vi "Actor Core.vi"(8 "error in":errorcluster, 11 "Sequence Controller in":refnum<class "Sequence Controller.lvclass">) -> (0 "error out":errorcluster, 3 "Actor out":refnum<class "Actor.lvclass">)   [LabVIEW 2018, in "Sequence Controller.lvclass"]
doc: "(<B>Filename</B>: Actor Framework.lvlib:Actor.lvclass:Actor Core.vi)\n\nReceives messages to the actor, reacts to them, and initiates any error handling that may shut the actor down.\n\nDescendant classes may override this VI to append parallel tasks for the actor to complete while it handles messages. Overrides use the Call Parent Method node."
uses:
  Sequence Controller.lvclass
  C:/github/LabActor/Sequence Elements/Sequence Element/Sequence Element.lvclass
  C:/github/LabActor/Template Module/Template Module.lvclass
  C:/Program Files/National Instruments/LabVIEW 2018/vi.lib/ActorFramework/Actor/Actor.lvclass
  <vilib>/ActorFramework/Actor/Actor.lvclass
  Sequence Controller.lvclass/Sequence Controller.ctl
  Template Module/Template Module.lvclass/Template Module.ctl
  <vilib>/ActorFramework/Actor/Actor.lvclass/Actor.ctl
  <vilib>/ActorFramework/Message Enqueuer/Message Enqueuer.lvclass/Message Enqueuer.ctl
  Sequence Elements/Sequence Element Messages/Items Mouse Click Msg/Items Mouse Click Msg.lvclass/Items Mouse Click Msg.ctl
  Application Controller Messages/Launch Object by Type Msg/Launch Object by Type Msg.lvclass/Launch Object by Type Msg.ctl
  Sequence Controller Messages/Remove Sequence Element Msg/Remove Sequence Element Msg.lvclass/Remove Sequence Element Msg.ctl
  Template Module Messages/Open Item Msg/Open Item Msg.lvclass/Open Item Msg.ctl
  Template Module/Read stop event.vi
  Template Module/Read Name.vi
  <vilib>/ActorFramework/Message Enqueuer/Init from Existing Queue.vi
  <vilib>/ActorFramework/Message Enqueuer/Enqueue.vi
  Sequence Elements/Sequence Element Messages/Items Mouse Click Msg/Items Mouse Click Msg.lvclass
  C:/Program Files/National Instruments/LabVIEW 2018/vi.lib/ActorFramework/Message/Message.lvclass
  Application Controller Messages/Launch Object by Type Msg/Launch Object by Type Msg.lvclass
  Sequence Controller Messages/Remove Sequence Element Msg/Remove Sequence Element Msg.lvclass
  Template Module Messages/Open Item Msg/Open Item Msg.lvclass
  <vilib>/ActorFramework/Message Priority Queue/Priority Enqueue.vi
  <vilib>/ActorFramework/Message Enqueuer/Message Enqueuer.lvclass
  Process Controller/Process Controller.lvclass
panel:
  in  "Remove Button":bool
  in  "Add Button":bool
  in  "Items":i32(listbox)
  in  "Measure sequence":string(tree)
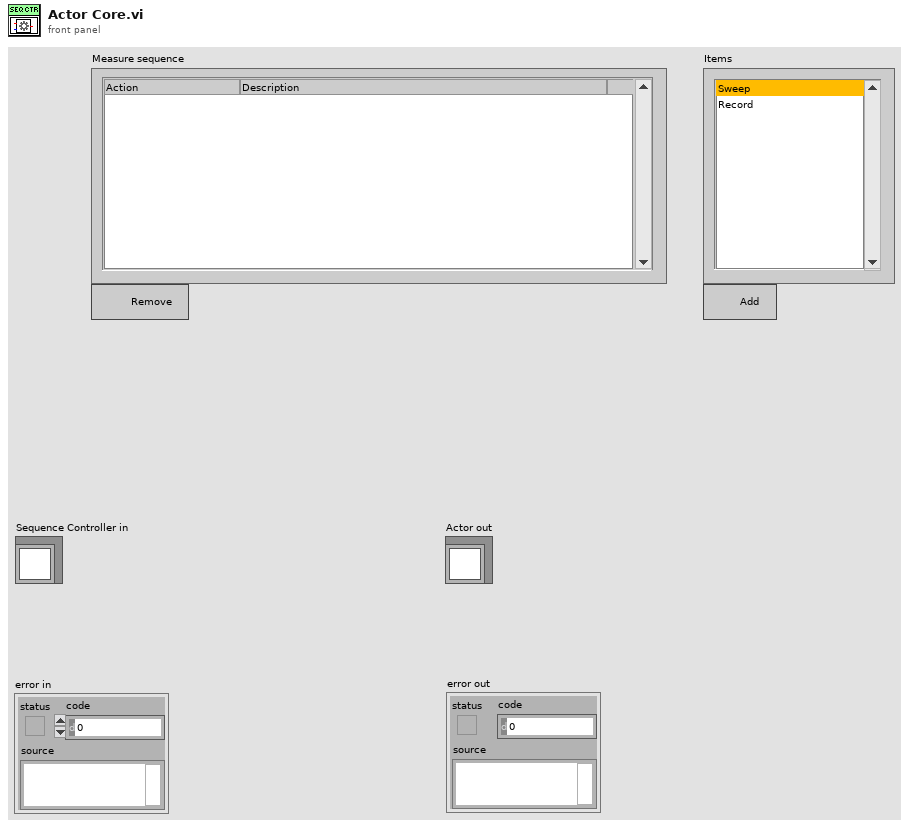
[diagram p1: front panel]
types:
  T1 = typedef "imagedata.ctl" = cluster{"image type":i32, "image depth":i32, "image":u8[], "mask":u8[], "colors":u32[], "Rectangle":cluster{"left":i16, "top":i16, "right":i16, "bottom":i16}}
  T2 = typedef "LVPoint32TypeDef.ctl" = cluster{"Horizontal":i32, "Vertical":i32}
  T3 = cluster{"Shift":bool, "Ctrl":bool, "Alt":bool, "Cmd":bool, "Opt":bool}
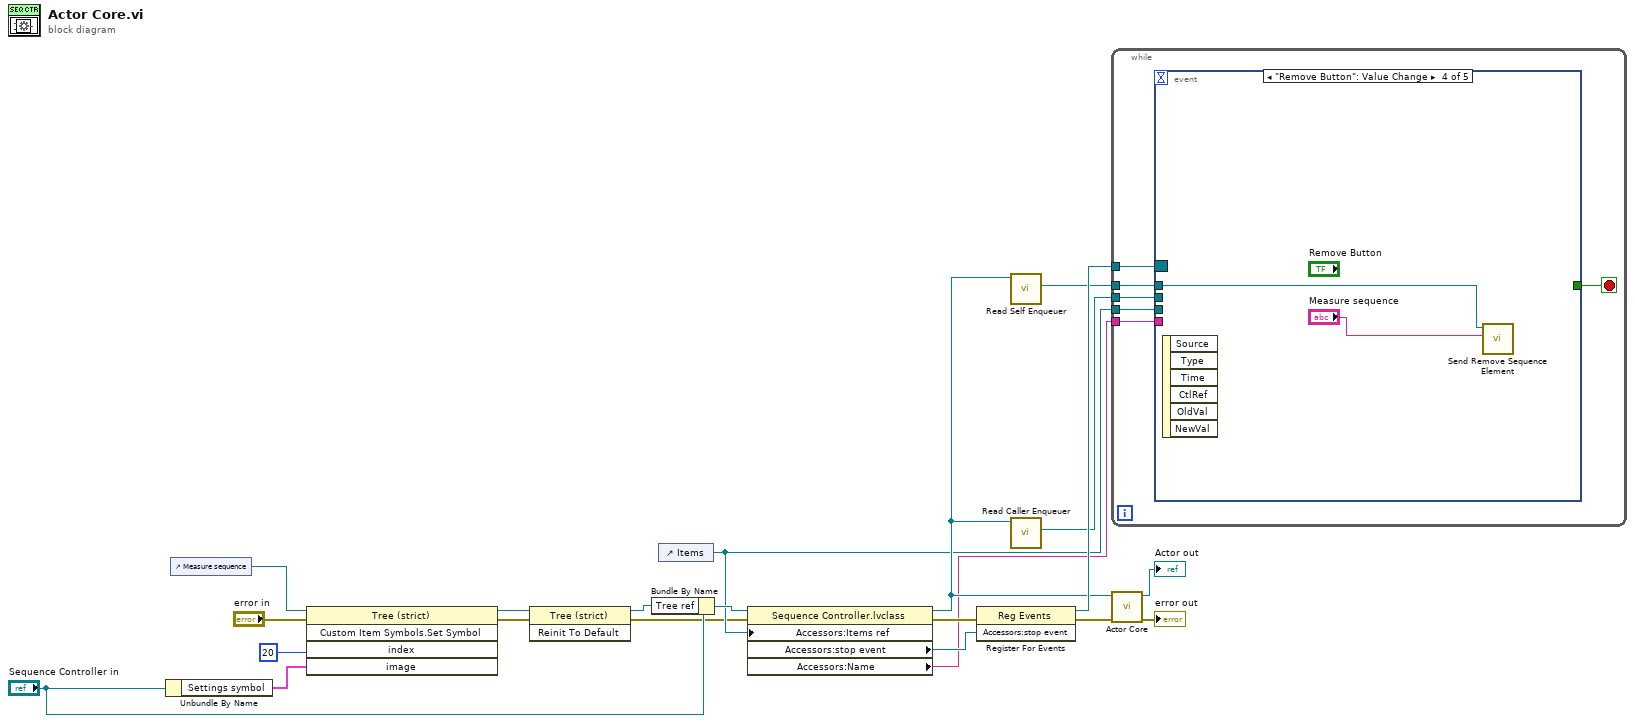
[diagram p0: block diagram]
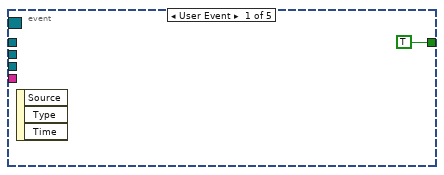
[diagram p2: hidden frame]
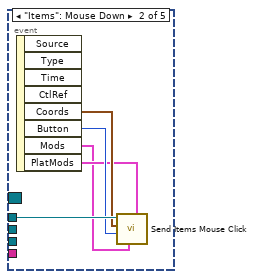
[diagram p3: hidden frame]
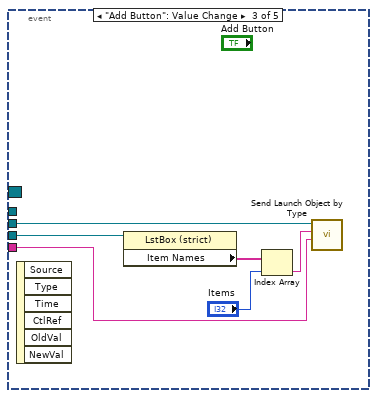
[diagram p4: hidden frame]
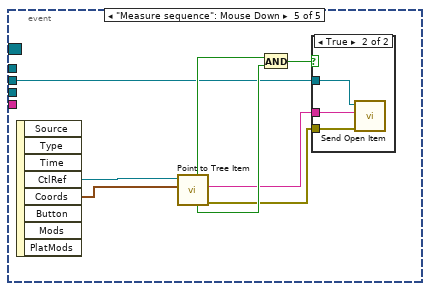
[diagram p5: hidden frame]
diagram:
  n1 = Unbundle By Name("Sequence Controller in") -> ("Settings symbol"=w10:T1)
  n2 = control-ref of="Measure sequence"() -> (w14:refnum<vi>)
  n3 = invoke class="Tree (strict)" method="Custom Item Symbols.Set Symbol"(reference=w14, error in="error in", "index"=20 ("Index"), "image"=w10) -> (reference out=w4:refnum<vi>, error out=w2:errorcluster)  [unwired: 1 in, 3 out]
  n4 = invoke class="Tree (strict)" method="Reinit To Default"(reference=w4, error in=w2) -> (reference out=w3:refnum<vi>, error out=w1:errorcluster)  [unwired: 1 in, 1 out]
  n5 = Bundle By Name(cluster="Sequence Controller in", "Tree ref"=w3) -> (w15:refnum<class "Sequence Controller.lvclass">)
  n6 = control-ref of="Items"() -> (w6:refnum<vi>)
  n7 = property class="Sequence Controller.lvclass"(reference=w15, error in=w1, "Accessors:Items ref"=w6) -> (reference out=w8:refnum<class "Sequence Controller.lvclass">, error out=w18:errorcluster, "Accessors:stop event"=w9:refnum<user-event>, "Accessors:Name"=w5:string)
  n8 = register-events(error in=w18, w9) -> (reference out=w19:refnum<event-registration>, error out=w17:errorcluster)  [unwired: 1 in]
  n9 = call <vilib>:"Read Self Enqueuer.vi"("Actor"=w8) -> ("Self Enqueuer"=w16:refnum<class "Message Enqueuer.lvclass">)  [unwired: 10 in]
  n10 = call <vilib>:"Read Caller Enqueuer.vi"("Actor"=w8) -> ("Caller Enqueuer"=w7:refnum<class "Message Enqueuer.lvclass">)  [unwired: 10 in]
  n11 = while {
    tunnel: w19 -> [w27]
    tunnel: w16 -> [w25]
    tunnel: w7 -> [w24]
    tunnel: w6 -> [w23]
    tunnel: w5 -> [w22]
    stop <- w26 stop-if-true
    n12 = event shown="[3] \"Remove Button\": Value Change" {
      selector: w27 -> [_ _ _ _ _]
      dyn-events: _ -> [_ _ _ _ _]
      timeout: _ -> [_ _ _ _ _]
      tunnel: [TRUE _ _ _ _] -> w26
      tunnel: w25 -> [_ w33 _ w41 _]
      tunnel: w24 -> [_ _ w34 _ w44]
      tunnel: w23 -> [_ _ w39 _ _]
      tunnel: w22 -> [_ _ w36 _ _]
      event User Event {
        n13 = event-data() -> ()  [unwired: 1 in, 3 out]
      }
      event "Items": Mouse Down {
        n14 = event-data() -> ("Coords"=w32:T2, "Button"=w31:u16, "Mods"=w29:cluster{"Double Click":bool, "Menu Key":bool}, "PlatMods"=w30:T3)  [unwired: 1 in, 4 out]
        n15 = call "Send Items Mouse Click.vi"("PlatMods"=w30, "Mods"=w29, "Button"=w31, "Coords"=w32, "Message Enqueuer"=w33) -> ()  [unwired: 5 in, 2 out]
      }
      event "Add Button": Value Change {
        n16 = event-data() -> ()  [unwired: 1 in, 6 out]
        n17 = property class="LstBox (strict)"(reference=w39) -> ("Item Names"=w38:string[])  [unwired: 1 in, 2 out]
        n18 = Index Array(array=w38, index="Items") -> (element=w35:string)
        n19 = call "Send Launch Object by Type.vi"("Requestor"=w36, "Type"=w35, "Message Enqueuer"=w34) -> ()  [unwired: 7 in, 2 out]
      }
      event "Remove Button": Value Change {
        n20 = event-data() -> ()  [unwired: 1 in, 6 out]
        n21 = call "Send Remove Sequence Element.vi"("Name"="Measure sequence", "Message Enqueuer"=w41) -> ()  [unwired: 8 in, 2 out]
      }
      event "Measure sequence": Mouse Down {
        n22 = event-data() -> ("CtlRef"=w49:refnum<vi>, "Coords"=w48:T2)  [unwired: 1 in, 6 out]
        n23 = call "Point to Tree Item.vi"("Coords"=w48, "reference"=w49) -> ("Error Out"=w42:errorcluster, "Item"=w43:string, "In Symbol?"=w46:bool, "Valid"=w47:bool)  [unwired: 5 in, 1 out]
        n24 = And(x=w47, y=w46) -> (x .and. y?=w45:bool)
        n25 = case shown="True" w45 {
          tunnel: w44 -> [_ w52]
          tunnel: w43 -> [_ w51]
          tunnel: w42 -> [_ w50]
          frame False {
          }
          frame True {
            n26 = call "Send Open Item.vi"("error in (no error)"=w50, "Item name"=w51, "Message Enqueuer"=w52) -> ()  [unwired: 7 in, 2 out]
          }
        }
      }
    }
  }
  n27 = call-parent "Actor Core.vi"("error in"=w17, "Measure Object in"=w8) -> ("error out"=→"error out":errorcluster, "Actor out"=→"Actor out":refnum<class "Actor.lvclass">)  [unwired: 8 in]
